vi "Build Error Message.vi"(8 "error in (no error)":errorcluster, 10 "Data":variant, 11 "Arg":string) -> (0 "error out":errorcluster)   [LabVIEW 2020, in "Code Cleanup.lvlib" / "FaKI State Machine.lvlib"]
doc: "Appends text to the end of the error message indicating the State/Arg where the error occurred, and works in conjunction with <B>Producer Loop Guard Clause.vi</B> to catch and handle any errors that may have occurred in the Producer Loop."
uses:
  FaKI State Machine.lvlib
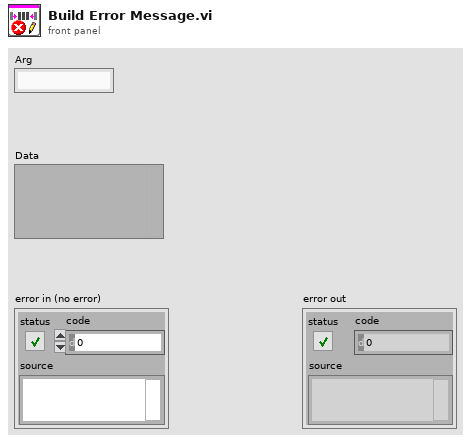
[diagram p1: front panel]
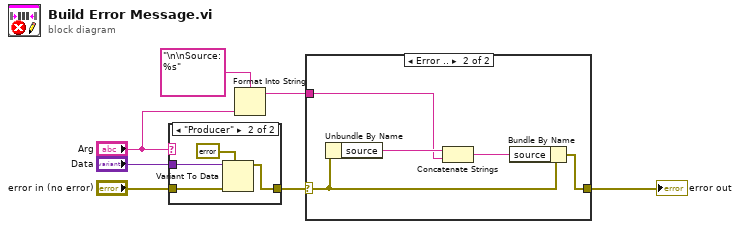
[diagram p0: block diagram]
diagram:
  n1 = case shown="\"Producer\"" "Arg" {
    tunnel: "Data" -> [_ w11]
    tunnel: "error in (no error)" -> [w8 w12]
    tunnel: [w8 w9] -> w3
    frame "", Default {
    }
    frame "Producer" {
      n2 = Variant To Data(error in=w12, type=errorcluster {"status"=FALSE, "code"=0, "source"=""} ("error out"), Variant=w11) -> (data=w9:errorcluster)  [unwired: 1 out]
    }
  }
  n3 = Format Into String(format string="\n\nSource: %s", "Arg") -> (resulting string=w2:string)  [unwired: 2 in, 1 out]
  n4 = case shown="Error .." w3 {
    selector: w3 -> [w13 w18]
    tunnel: [w13 w17] -> w1
    tunnel: w2 -> [_ w14]
    frame No Error {
    }
    frame Error {
      n5 = Unbundle By Name(w18) -> ("source"=w16:string)
      n6 = Concatenate Strings(w16, w14) -> (w15:string)
      n7 = Bundle By Name(cluster=w18, "source"=w15) -> (w17:errorcluster)
    }
  }
  "error out" <- w1
